vi "Actor Core.vi"(8 "error in":errorcluster, 11 "Nested in":refnum<class "Doña Rata Actor.lvclass">) -> (0 "error out":errorcluster, 3 "Actor out":refnum<class "Actor.lvclass">)   [LabVIEW 2020, in "Doña Rata Actor.lvlib" / "Doña Rata Actor.lvclass"]
doc: "(<B>Filename</B>: Actor Framework.lvlib:Actor.lvclass:Actor Core.vi)\n\nReceives messages to the actor, reacts to them, and initiates any error handling that may shut the actor down.\n\nDescendant classes may override this VI to append parallel tasks for the actor to complete while it handles messages. Overrides use the Call Parent Method node."
uses:
  C:/Program Files/National Instruments/LabVIEW 2020/vi.lib/ActorFramework/Actor/Actor.lvclass
  <vilib>/ActorFramework/Actor/Actor.lvclass
  <vilib>/ActorFramework/Actor/Actor.lvclass/Actor.ctl
  <vilib>/ActorFramework/Message Enqueuer/Message Enqueuer.lvclass/Message Enqueuer.ctl
  <vilib>/ActorFramework/Message Enqueuer/Init from Existing Queue.vi
  <vilib>/ActorFramework/Message Enqueuer/Enqueue.vi
  <vilib>/ActorFramework/Stop Msg/Stop Msg.lvclass
  C:/Program Files/National Instruments/LabVIEW 2020/vi.lib/ActorFramework/Message/Message.lvclass
  <vilib>/ActorFramework/Message Priority Queue/Priority Enqueue.vi
  <vilib>/ActorFramework/Message Enqueuer/Message Enqueuer.lvclass
panel:
  in  "Productos":i32(listbox)
  in  "Comprar":bool
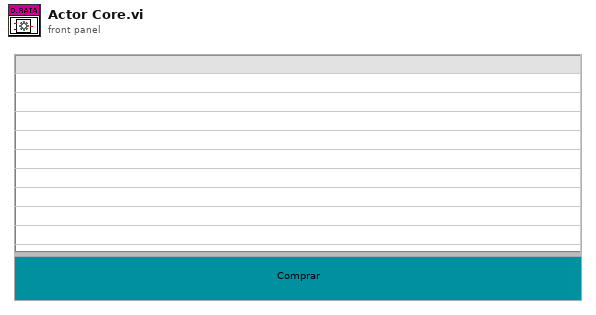
[diagram p1: front panel]
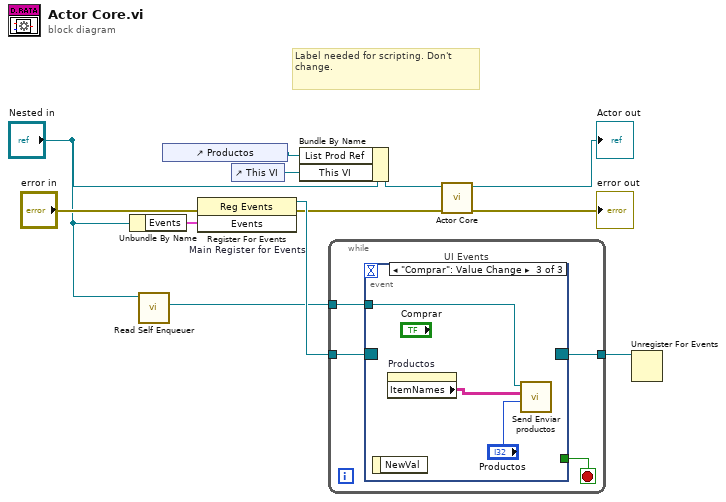
[diagram p0: block diagram]
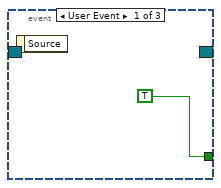
[diagram p2: hidden frame]
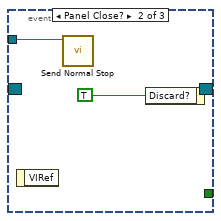
[diagram p3: hidden frame]
diagram:
  # "Label needed for scripting. Don't change."
  n1 = Unbundle By Name("Nested in") -> ("Events"=w9:cluster{"Stop":refnum<user-event>})
  n2 = call <vilib>:"Read Self Enqueuer.vi"("Actor"="Nested in") -> ("Self Enqueuer"=w7:refnum<class "Message Enqueuer.lvclass">)  [unwired: 10 in]
  n3 = control-ref of="Productos"() -> (w1:refnum<vi>)
  n4 = register-events "Main Register for Events"(error in="error in", w9) -> (reference out=w10:refnum<event-registration>, error out=w5:errorcluster)  [unwired: 1 in]
  n5 = control-ref of="This VI"() -> (w2:refnum<vi>)
  n6 = Bundle By Name(cluster="Nested in", "List Prod Ref"=w1, "This VI"=w2) -> (w3:refnum<class "Doña Rata Actor.lvclass">)
  n7 = while {
    tunnel: w10 -> [w16]
    tunnel: [w14] -> w8
    tunnel: w7 -> [w13]
    stop <- w15 stop-if-true
    n8 = event "UI Events" shown="[2] \"Comprar\": Value Change" {
      selector: w16 -> [_ _ _]
      dyn-events: [_ _ _] -> w14
      timeout: _ -> [_ _ _]
      tunnel: [TRUE _ _] -> w15
      tunnel: w13 -> [_ w18 w21]
      event User Event {
        n9 = event-data() -> ()  [unwired: 1 in, 1 out]
      }
      event Panel Close? {
        n10 = event-data() -> ()  [unwired: 1 in, 1 out]
        n11 = call <vilib>:"Send Normal Stop.vi"("Message Enqueuer"=w18) -> ()  [unwired: 10 in, 1 out]
        n12 = event-data("Discard?"=TRUE) -> ()  [unwired: 1 in, 1 out]
      }
      event "Comprar": Value Change {
        n13 = event-data() -> ()  [unwired: 1 in, 1 out]
        n14 = property on="Productos" class="MCListbox (strict)"() -> ("ItemNames"=w20:string[][])  [unwired: 2 in, 2 out]
        n15 = call "Send Enviar productos.vi"("index"="Productos", "Item names"=w20, "Message Enqueuer"=w21) -> ()  [unwired: 7 in, 2 out]
      }
    }
  }
  n16 = call-parent "Actor Core.vi"("error in"=w5, "Actor in"=w3) -> ("error out"=→"error out":errorcluster, "Actor out"=→"Actor out":refnum<class "Actor.lvclass">)  [unwired: 8 in]
  n17 = Unregister For Events(event registration refnum=w8) -> ()  [unwired: 1 in, 1 out]
